vi "getFilePattern.vi"(8 "error in (no error)":errorcluster, 11 "Document in":refnum<class "Document.lvclass">) -> (0 "error out":errorcluster, 1 "pattern":string, 2 "pattern label":string, 3 "Document out":refnum<class "Document.lvclass">)   [LabVIEW 2020, in "LabVIEW NPOI.lvlib" / "Document.lvclass"]
doc: "Private method to get the <b>pattern lable</b> and the <b>pattern</b> from the <b>Docuement</b>.\n\nNote: \n<b>pattern lable</b>: is the label to display in the file dialog box next to the custom pattern.\n<b>pattern</b>: restricts the files displayed in the dialog box to those whose name matches pattern."
uses:
  Document.lvclass
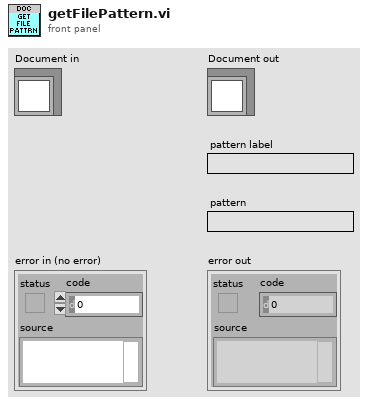
[diagram p1: front panel]
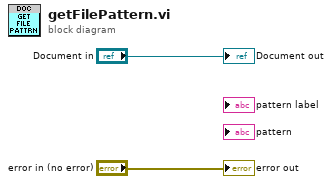
[diagram p0: block diagram]
diagram:
  "error out" <- "error in (no error)"
  "Document out" <- "Document in"
